vi "Baysian_LDA.vi"(4 "nontarget_order":i32[][](array[numeric]), 6 "target_order":i32[](array[numeric]), 7 "RAW__EEG(brain.txt)":dbl[][](array[numeric]), 8 "Target_ERP":dbl[][](array[numeric]), 10 "Nontarget_ERP":dbl[][](array[numeric]), 11 "prior_LDA":T1) -> (0 "Weight_vector":dbl[](array[numeric]), 1 "Nontarget_Weighted_ERP":dbl[][](array[numeric]), 2 "Target_Weighted_ERP":dbl[][](array[numeric]), 3 "Bayseian_LDA":T1)   [LabVIEW 2013]
uses:
  <vilib>/Analysis/Matrix/Datatypes/RealMatrix.ctl
  <vilib>/Analysis/baseanly.llb/Real A x B.vi
  <vilib>/Analysis/Matrix/Numeric/Conversions/Array To Matrix - RA2.vi
  <vilib>/Analysis/Matrix/Numeric/Conversions/Array To Matrix - RA.vi
  <vilib>/Analysis/Matrix/Numeric/Conversions/Matrix To Array - RM.vi
  <vilib>/Analysis/Matrix/Numeric/Subtract/Subtract - RM,RM.vi
  <vilib>/Analysis/Matrix/Numeric/Absolute Value/Absolute Value - RM.vi
  <vilib>/Analysis/Matrix/NI_Matrix.lvlib
  <vilib>/Analysis/NI_AALBase.lvlib
panel:
  # "INPUTS"
  # "OUTPUTS"
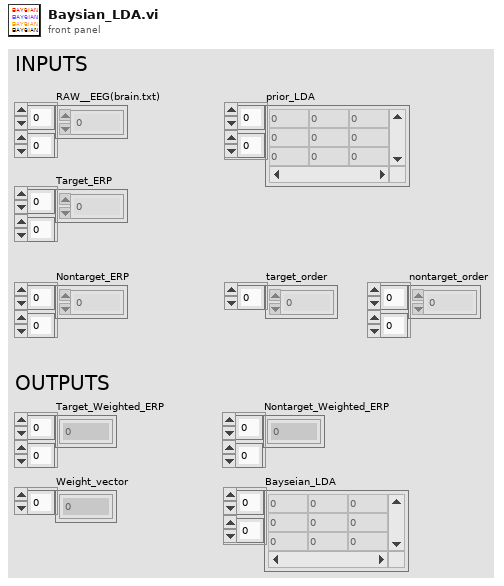
[diagram p1: front panel]
types:
  T1 = typedef "NI_Matrix.lvlib/RealMatrix.ctl" = dbl[][]
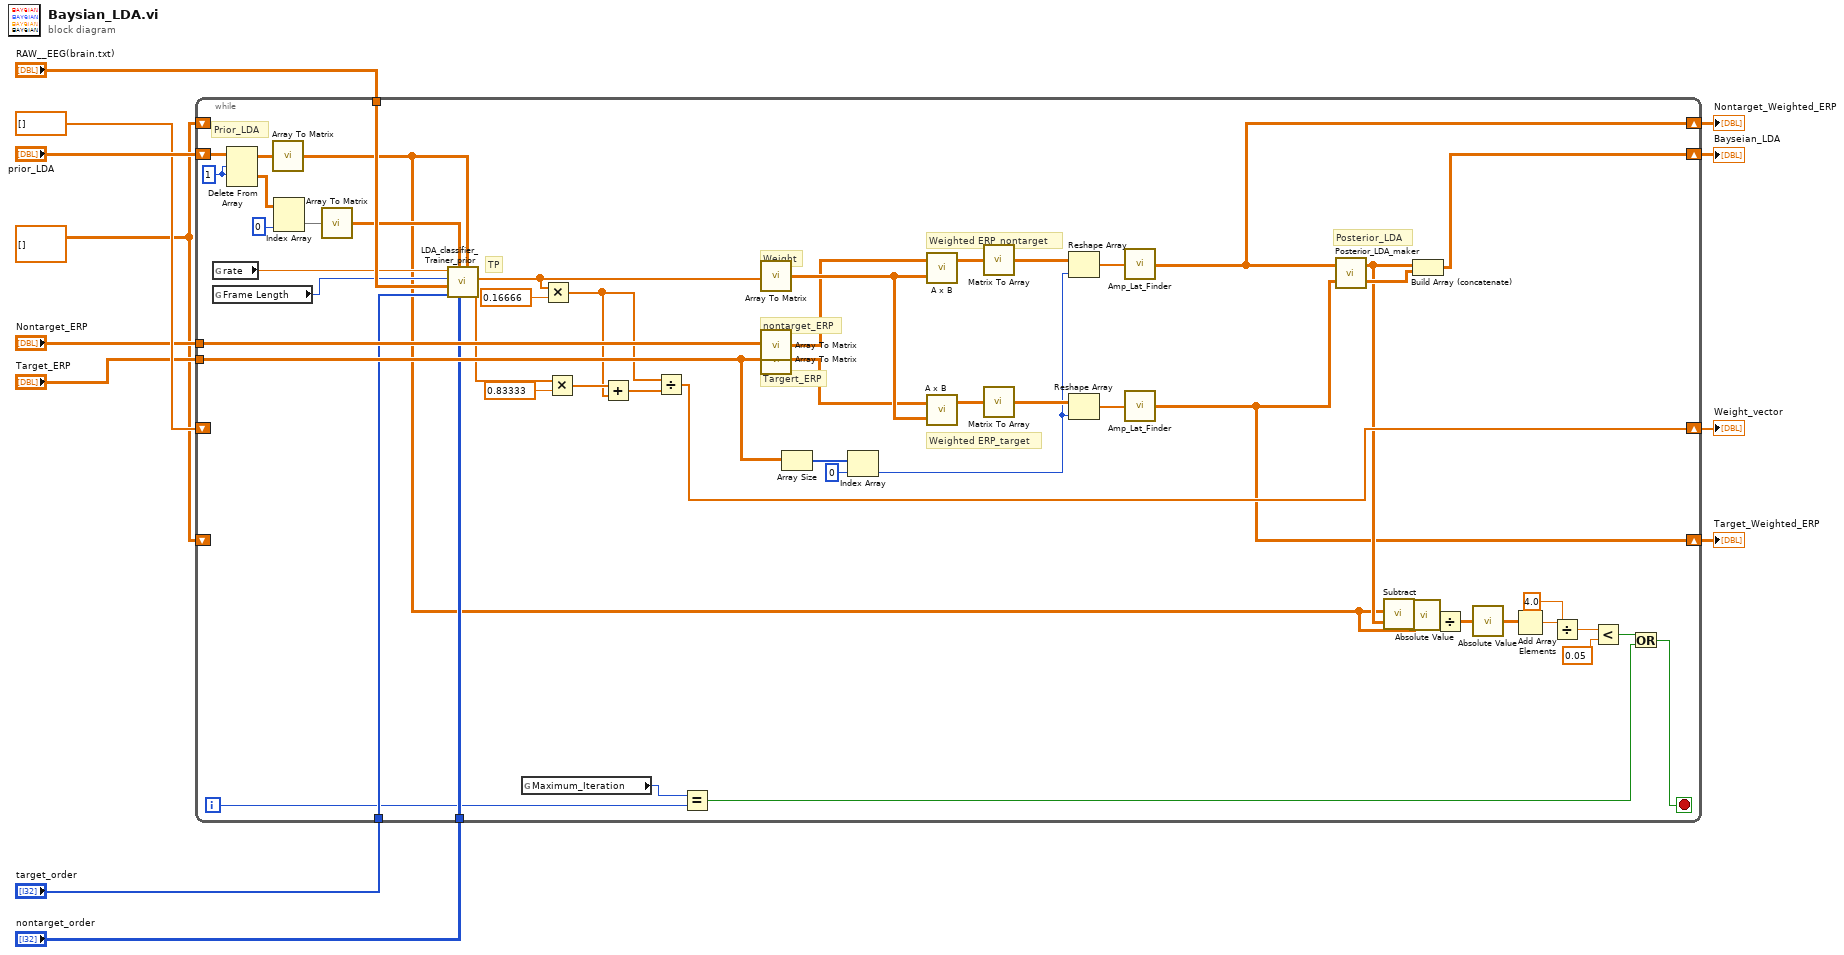
[diagram p0: block diagram]
diagram:
  w1 = dbl[][] [] ("Real 2D Array")
  n1 = while {
    tunnel: "Nontarget_ERP" -> [w61]
    tunnel: "Target_ERP" -> [w56]
    tunnel: "RAW__EEG(brain.txt)" -> [w52]
    tunnel: "target_order" -> [w49]
    shift-right: [w41] -> w4
    shift-left: "prior_LDA" -> [w43]
    tunnel: "nontarget_order" -> [w40]
    shift-right: [w14] -> w5
    shift-left: w1 -> [_]
    shift-right: [w13] -> w2
    shift-left: w1 -> [_]
    shift-right: [w30] -> w3
    shift-left: dbl[] [] ("Real 2D Array") -> [_]
    i -> [w29]
    stop <- w15 stop-if-true
    w45 = 1 ("인덱스 (행)")
    # "Posterior_LDA"
    # "Prior_LDA"
    # "TP"
    # "Targert_ERP"
    # "nontarget_ERP"
    # "Weighted ERP_target"
    # "Weighted ERP_nontarget"
    # "Weight"
    n2 = global read "Control_Panel.vi" "rate"() -> (w51:dbl)
    n3 = global read "Control_Panel.vi" "Frame Length"() -> (w50:i32)
    n4 = Delete From Array(array=w43, length=w45, index (row)=w45) -> (deleted portion=w48:T1, array with subset deleted=w47:T1)  [unwired: 1 in]
    n5 = call-poly <vilib>:"Array To Matrix.vi"("Real 2D Array"=w47) -> ("Real Matrix"=w24:T1)
    n6 = Index Array(array=w48, index (col)=0 ("인덱스")) -> (element=w46:dbl[])  [unwired: 1 in]
    n7 = call-poly <vilib>:"Array To Matrix.vi"("Real 1D Array"=w46) -> ("Real Matrix (Column Vector)"=w42:T1)
    n8 = call "LDA_classifier_Trainer_prior.vi"("Matrix"=w24, "Non_target_Flash_order"=w40, "Value"=w42, "Target_Flash_Order"=w49, "Brain_data_source"=w52, "samples per channel"=w50, "rate"=w51) -> ("FP"=w34:dbl[], "TP"=w36:dbl[])  [unwired: 3 in]
    n9 = global read "Control_Panel.vi" "Maximum_Iteration"() -> (w28:i64)
    n10 = Multiply(x=w36, y=0.16666) -> (x*y=w31:dbl[])
    n11 = Multiply(x=w34, y=0.83333) -> (x*y=w33:dbl[])
    n12 = Add(x=w33, y=w31) -> (x+y=w32:dbl[])
    n13 = Divide(x=w31, y=w32) -> (x/y=w30:dbl[])
    n14 = Equal?(x=w28, y=w29) -> (x = y?=w16:bool)
    n15 = call-poly <vilib>:"Array To Matrix.vi"("Real 1D Array"=w36) -> ("Real Matrix (Column Vector)"=w64:T1)
    n16 = call-poly <vilib>:"Array To Matrix.vi"("Real 2D Array"=w61) -> ("Real Matrix"=w60:T1)
    n17 = call-poly <vilib>:"Array To Matrix.vi"("Real 2D Array"=w56) -> ("Real Matrix"=w59:T1)
    n18 = Array Size(array=w56) -> (size(s)=w55:i32[])
    n19 = Index Array(array=w55, index=0) -> (element=w53:i32)
    n20 = call-poly <vilib>:"A x B.vi"("B"=w64, "A"=w60) -> ("A x B"=w63:T1)  [unwired: 1 out]
    n21 = call-poly <vilib>:"A x B.vi"("B"=w64, "A"=w59) -> ("A x B"=w62:T1)  [unwired: 1 out]
    n22 = call-poly <vilib>:"Matrix To Array.vi"("Real Matrix"=w63) -> ("Real 2D Array"=w58:dbl[][])
    n23 = call-poly <vilib>:"Matrix To Array.vi"("Real Matrix"=w62) -> ("Real 2D Array"=w57:dbl[][])
    n24 = Reshape Array(w58, w53) -> (w39:dbl[])
    n25 = Reshape Array(w57, w53) -> (w38:dbl[])
    n26 = call "Amp_Lat_Finder.vi"("ERP_vector"=w39) -> ("LDA_Parameter"=w14:dbl[][])
    n27 = call "Amp_Lat_Finder.vi"("ERP_vector"=w38) -> ("LDA_Parameter"=w13:dbl[][])
    n28 = call "Posterior_LDA_maker.vi"("Target_LDA_Parameter"=w13, "Nontarget_LDA_Parameter"=w14) -> ("A * B 2"=w65:T1, "A * B"=w27:T1)
    n29 = call-poly <vilib>:"Subtract.vi"("Real Matrix B"=w27, "Real Matrix A"=w24) -> ("A - B"=w26:T1)
    n30 = call-poly <vilib>:"Absolute Value.vi"("Real Matrix A"=w26) -> ("|A|"=w25:T1)
    n31 = Build Array (concatenate)(w27, w65) -> (w41:T1)
    n32 = Divide(x=w25, y=w24) -> (x/y=w23:T1)
    n33 = call-poly <vilib>:"Absolute Value.vi"("Real Matrix A"=w23) -> ("|A|"=w22:T1)
    n34 = Add Array Elements(numeric array=w22) -> (sum=w21:dbl)
    n35 = Divide(x=w21, y=4.0) -> (x/y=w19:dbl)
    n36 = Less?(x=w19, y=0.05) -> (x < y?=w17:bool)
    n37 = Or(x=w17, y=w16) -> (x .or. y?=w15:bool)
  }
  "Nontarget_Weighted_ERP" <- w5
  "Bayseian_LDA" <- w4
  "Weight_vector" <- w3
  "Target_Weighted_ERP" <- w2
